vi "removeVirtualDrive.vi"(8 "error in (no error)":errorcluster, 11 "BuildWorker Controller in":refnum<class "BuildWorker Controller.lvclass">) -> (0 "error out":errorcluster, 3 "BuildWorker Controller out":refnum<class "BuildWorker Controller.lvclass">)   [LabVIEW 2017, in "BuildWorker Interface.lvlib" / "BuildWorker Controller.lvclass"]
uses:
  BuildWorker Controller.lvclass
  BuildWorker Controller.lvclass/BuildWorker Controller.ctl
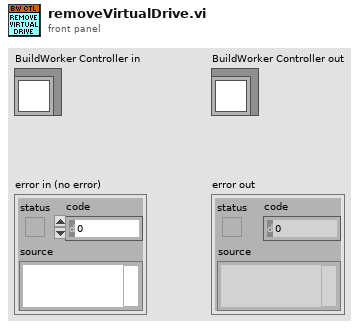
[diagram p1: front panel]
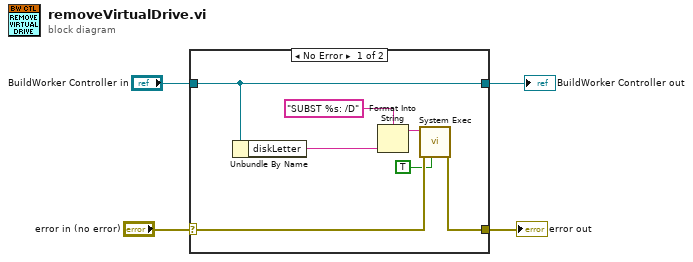
[diagram p0: block diagram]
diagram:
  n1 = case shown="No Error" "error in (no error)" {
    selector: "error in (no error)" -> [w7 w13]
    tunnel: [w6 w13] -> w1
    tunnel: [w11 w12] -> w3
    tunnel: "BuildWorker Controller in" -> [w11 w12]
    frame No Error {
      n2 = Unbundle By Name(w11) -> ("diskLetter"=w10:string)
      n3 = Format Into String(format string="SUBST %s: /D", w10) -> (resulting string=w8:string)  [unwired: 2 in, 1 out]
      n4 = call <vilib>:"System Exec.vi"("run minimized? (F)"=TRUE, "error in (no error)"=w7, "command line"=w8) -> ("error out"=w6:errorcluster)  [unwired: 5 in, 3 out]
    }
    frame Error {
    }
  }
  "error out" <- w1
  "BuildWorker Controller out" <- w3
